vi "Robot Global Data.vi"() -> ()   [LabVIEW 2015]
doc: "This global VI can contain as many global variables as you need. Place a control on the panel, give it a good name. To read or write to it from a VI, drag the icon to the diagram of that VI. You can also drag from the project. Click on the node to change which global you access. You shouldn't have multiple locations writing to a global or it will cause a race-condition."
uses:
  <vilib>/Rock Robotics/WPI/Camera/WPI_CameraImageSize.ctl
  <vilib>/Rock Robotics/WPI/DriverStation/WPI_DriverStationRobotMode2.ctl
  Type Defs/Shooter State.ctl
panel:
  in  "LB Trigger":bool
  in  "Button 3":bool
  in  "Finished Porticullis crossing":bool
  in  "Auto Crossing Finished":bool
  out "Auto Angle error":dbl
  out "Auto Left":dbl
  out "Auto Right":dbl
  out "Auto Angle":dbl
  out "Porticullis drivetrain control":dbl
  out "Crossing Porticullis?":bool
  out "Left Wheels tele":dbl
  out "Right Wheels tele":dbl
  in  "Start Button":bool
  in  "Button 0":bool
  out "Distance":dbl
  in  "Reset Grayhill":bool
  in  "Shooter State":T1
  out "YRPHfH":T2
  in  "B Button":bool
  in  "RB Trigger":bool
  in  "LB Button":bool
  in  "X Button":bool
  in  "Y Button":bool
  in  "A Button":bool
  out "Arm Setpoint":dbl
  out "Wheel Current Speed":dbl
  out "Ball In Shooter?":bool
  out "Ball In Intake?":bool
  out "Arm Current Position":dbl
  out "Arm Up?":bool
  in  "Robot Mode":T3
  in  "image size":T4=enum."320x240"
  in  "Enable Vision":bool
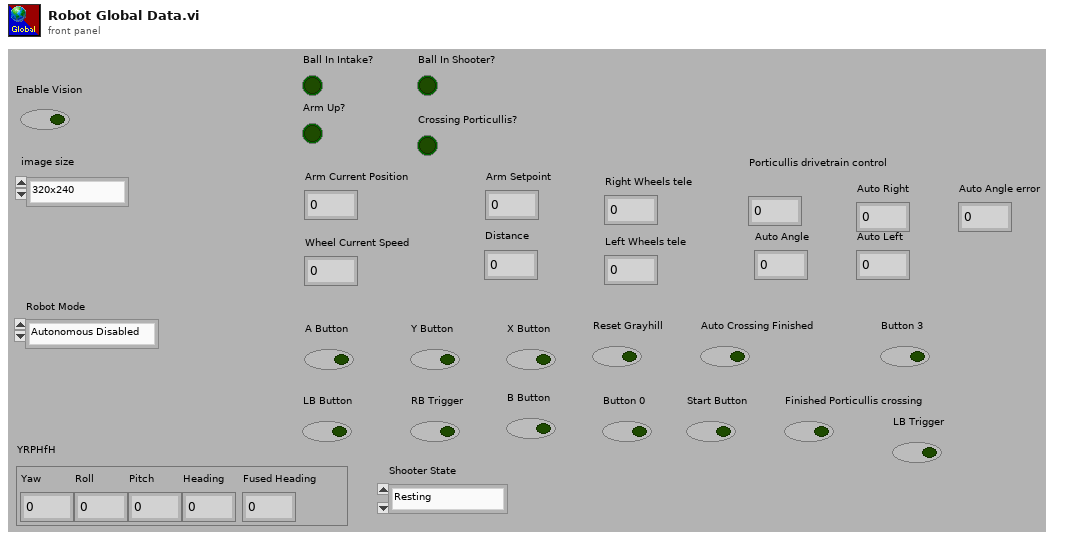
[diagram p1: front panel]
types:
  T1 = typedef "Shooter State.ctl" = enum16{"Resting", "Start Shooter", "Shooooot!"}
  T2 = cluster{"Yaw":dbl, "Roll":dbl, "Pitch":dbl, "Heading":dbl, "Fused Heading":dbl}
  T3 = typedef "WPI_DriverStationRobotMode2.ctl" = enum16{"Autonomous Disabled", "Autonomous Enabled", "Teleop Disabled", "Teleop Enabled", "Disconnected", "Finish", "Test Disabled", "Test Enabled", "Emergency Stopped"}
  T4 = typedef "WPI_CameraImageSize.ctl" = enum16{"640x480", "320x240", "160x120", "Custom"}
diagram:
